vi "Add Menu Items.vi"(7 "Menu control":T1=enum."Pulse", 8 "error in (no error)":errorcluster, 9 "Reset":bool, 10 "Item Names":string[](array[string]), 11 "Monitor-Pulse in":refnum<class "LabActor.lvclass">) -> (0 "error out":errorcluster, 3 "Monitor-Pulse out":refnum<class "LabActor.lvclass">)   [LabVIEW 2024, in "LabActor.lvclass"]
uses:
  LabActor.lvclass
  Controllers/Application Controller/Menu Control.ctl
  LabActor.lvclass/LabActor.ctl
  Controllers/Application Controller/Application Controller.lvclass
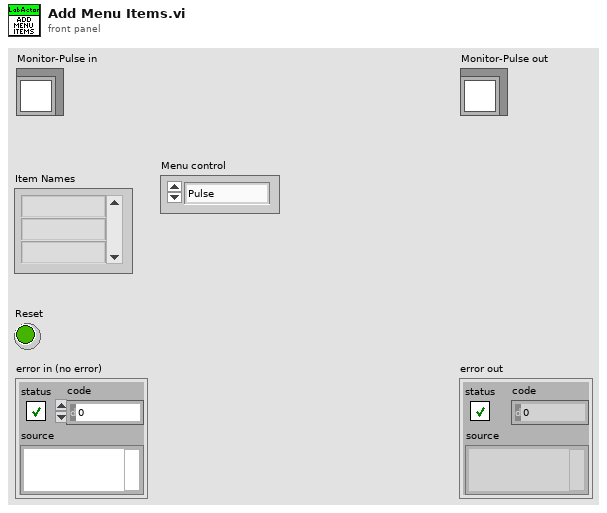
[diagram p1: front panel]
types:
  T1 = typedef "Menu Control.ctl" = enum16{"NONE", "Monitor", "Post-process", "Pulse"}
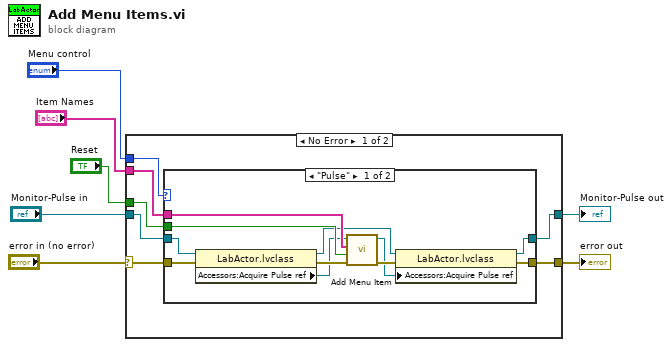
[diagram p0: block diagram]
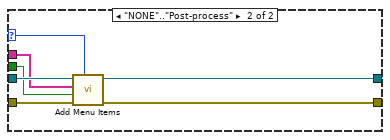
[diagram p2: hidden frame]
diagram:
  n1 = case shown="No Error" "error in (no error)" {
    selector: "error in (no error)" -> [w10 w34]
    tunnel: [w9 w34] -> w6
    tunnel: [w14 w33] -> w4
    tunnel: "Monitor-Pulse in" -> [w11 w33]
    tunnel: "Item Names" -> [w13 _]
    tunnel: "Reset" -> [w12 _]
    tunnel: "Menu control" -> [w8 _]
    frame No Error {
      n2 = case shown="\"Pulse\"" w8 {
        selector: w8 -> [_ w26]
        tunnel: [w16 w30] -> w14
        tunnel: w13 -> [w25 w29]
        tunnel: w12 -> [w24 w28]
        tunnel: w11 -> [w20 w32]
        tunnel: w10 -> [w23 w31]
        tunnel: [w17 w27] -> w9
        frame "Pulse" {
          n3 = property class="LabActor.lvclass"(reference=w20, error in=w23) -> (reference out=w19:refnum<class "LabActor.lvclass">, error out=w21:errorcluster, "Accessors:Acquire Pulse ref"=w18:refnum<vi>)
          n4 = call "Add Menu Item.vi"("error in (no error)"=w21, "Reset"=w24, "Item Names"=w25, "Queed Listbox ref"=w18) -> ("error out"=w22:errorcluster, "Queed Listbox ref out"=w15:refnum<vi>)  [unwired: 5 in, 1 out]
          n5 = property class="LabActor.lvclass"(reference=w19, error in=w22, "Accessors:Acquire Pulse ref"=w15) -> (reference out=w16:refnum<class "LabActor.lvclass">, error out=w17:errorcluster)
        }
        frame "NONE".."Post-process" {
          n6 = call-parent "Add Menu Items.vi"("Menu control"=w26, "error in (no error)"=w31, "Reset"=w28, "Item Names"=w29, "Application Controller in"=w32) -> ("error out"=w27:errorcluster, "Application Controller out"=w30:refnum<class "LabActor.lvclass">)  [unwired: 5 in]
        }
      }
    }
    frame Error {
    }
  }
  "error out" <- w6
  "Monitor-Pulse out" <- w4
